vi "Load meas device config.vi"(7 "Equipo a Utilizar":enum16{"SR830 Lock In", "TDS 2012B Osciloscope"}(ring), 8 "error in (no error)":errorcluster, 10 "Datos Adquisición":T1={"Equipo a Utilizar"=enum."TDS 2012B Osciloscope", "Montura"=enum."Zaber T-LSR450B", "Datos Zaber"={"Sentido de Adquisición"=TRUE, "Comenzar Desde Home?"=TRUE, "Distancia a recorrer (um)"=10.0, "Pasos motor"=0, "Distancia entre Lecturas (um)"=0.1, "Puerto"="UNKNOWN"}, "Datos Bipolar/Unipolar"={"Puerto COM"="UNKNOWN", "Pasos entre Lecturas"=0, "Numero de lecturas"=0, "Sentido del motor"=TRUE}, "Datos Archivo"={"Ruta Archivo"=path "", "Nombre de Prueba"=""}, "Datos actuales"={"Montura"="", "Equipo"="", "Posición Actual"="", "Distancia Total a recorrer"="", "distancia Entre lecturas"="", "Pasos entre lecturas"=""}, "Datos a Guardar In"={"Datos Cursor Tektronix"="", "Datos Lokin"="", "Posición Cero"=0.0, "Posición Actual"=0.0}, "Datos Osciloscopio"={"Sesión Visa Osciloscopio"="UNKNOWN", "Tipo de Adquisición"=enum."Voltaje Pico Pico", "Canal a Utilizar"=enum."Canal 1", "Parametros de Adquisición"=enum."Una Muestra", "Número Promedio"=2}, "Datos Lock In"={"Visa Lock in"="Tektronix_TDS2012C"}} {"Datos Osciloscopio"."Número Promedio" min=2 max=20; "Datos a Guardar In"."Posición Actual" format="%#_10f"; "Datos a Guardar In"."Posición Cero" format="%#_10f"; "Datos Bipolar/Unipolar"."Numero de lecturas" max=910098 step=1}, 11 "Refnum in":T7) -> (0 "error out":errorcluster, 2 "Datos Adquisición out":T1={"Equipo a Utilizar"=enum."TDS 2012B Osciloscope", "Montura"=enum."Zaber T-LSR450B", "Datos Zaber"={"Sentido de Adquisición"=FALSE, "Comenzar Desde Home?"=FALSE, "Distancia a recorrer (um)"=0.0, "Pasos motor"=0, "Distancia entre Lecturas (um)"=0.0, "Puerto"=""}, "Datos Bipolar/Unipolar"={"Puerto COM"="", "Pasos entre Lecturas"=0, "Numero de lecturas"=0, "Sentido del motor"=TRUE}, "Datos Archivo"={"Ruta Archivo"=path "", "Nombre de Prueba"=""}, "Datos actuales"={"Montura"="", "Equipo"="", "Posición Actual"="", "Distancia Total a recorrer"="", "distancia Entre lecturas"="", "Pasos entre lecturas"=""}, "Datos a Guardar In"={"Datos Cursor Tektronix"="", "Datos Lokin"="", "Posición Cero"=0.0, "Posición Actual"=0.0}, "Datos Osciloscopio"={"Sesión Visa Osciloscopio"="Tektronix_TDS2012C", "Tipo de Adquisición"=enum."Voltaje Pico Pico", "Canal a Utilizar"=enum."Canal 1", "Parametros de Adquisición"=enum."Una Muestra", "Número Promedio"=2}, "Datos Lock In"={"Visa Lock in"="Tektronix_TDS2012C"}} {"Datos Osciloscopio"."Número Promedio" min=2 max=20; "Datos a Guardar In"."Posición Actual" format="%#_10f"; "Datos a Guardar In"."Posición Cero" format="%#_10f"; "Datos Bipolar/Unipolar"."Numero de lecturas" max=910098 step=1}, 3 "Refnum out":T7)   [LabVIEW 2020]
uses:
  Type Definitions/datos osciloscopio.ctl
  <vilib>/Utility/config.llb/NI_LVConfig.lvlib
  <vilib>/Utility/config.llb/Read Key (String).vi
  <vilib>/Utility/config.llb/Read Key (U32).vi
  <vilib>/Utility/config.llb/Read Key (I32).vi
  <vilib>/Utility/config.llb/Config Data RefNum.ctl
  Type Definitions/Datos Zaber.ctl
  Type Definitions/parametros motores.ctl
  Type Definitions/Datos a Guardar.ctl
  H:/Mi unidad/Departamento de Ingenieria/Investigadores/Gabriel Ramos/Proyecto Monturas v13/LV Source/Type Definitions/Tipos de montura.ctl
  Type Definitions/Asistente de adquisicion Cluster.ctl
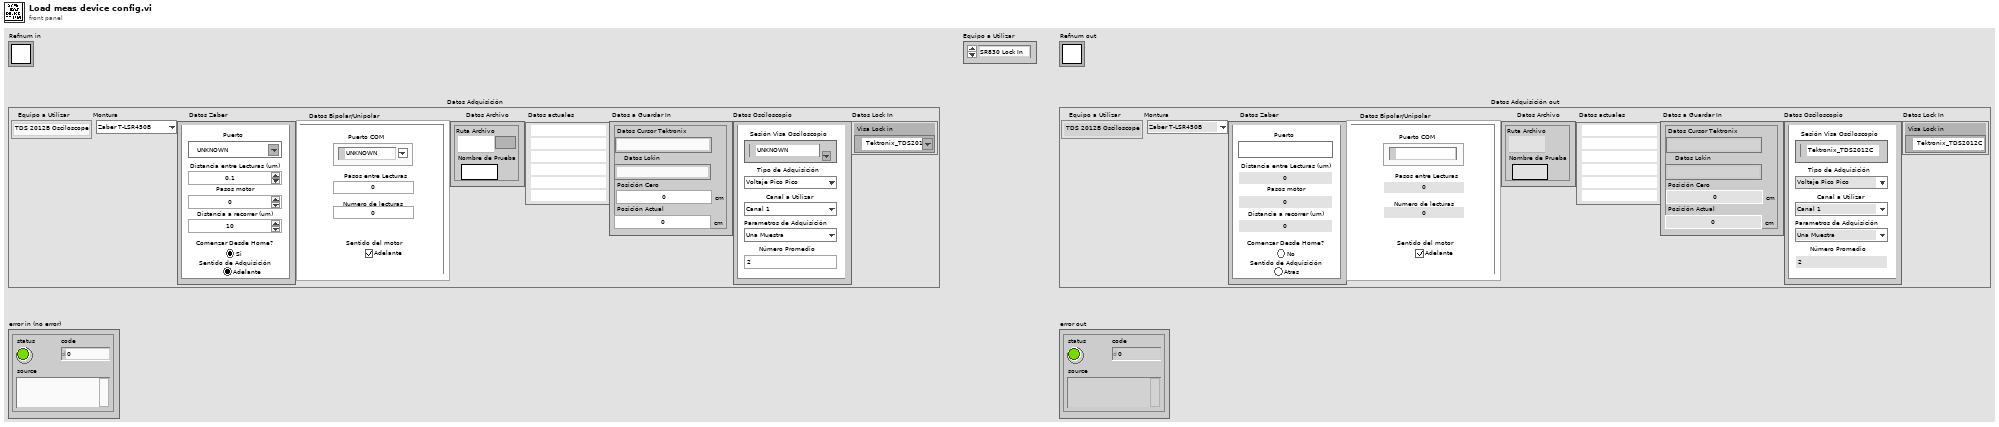
[diagram p1: front panel]
types:
  T1 = typedef "Asistente de adquisicion Cluster.ctl" = cluster{"Equipo a Utilizar":enum16{"SR830 Lock In", "TDS 2012B Osciloscope"}, "Montura":T2, "Datos Zaber":T3, "Datos Bipolar/Unipolar":T4, "Datos Archivo":cluster{"Ruta Archivo":path, "Nombre de Prueba":string}, "Datos actuales":cluster{"Montura":string, "Equipo":string, "Posición Actual":string, "Distancia Total a recorrer":string, "distancia Entre lecturas":string, "Pasos entre lecturas":string}, "Datos a Guardar In":T5, "Datos Osciloscopio":T6, "Datos Lock In":cluster{"Visa Lock in":refnum<visa-resource-name>}}
  T2 = typedef "Tipos de montura.ctl" = enum16{"Zaber T-LSR450B", "Zaber-T-LSR300B", "Zaber-T-LSRxxx", "Motor Bipolar", "Motor Unipolar"}
  T3 = typedef "Datos Zaber.ctl" = cluster{"Sentido de Adquisición":bool, "Comenzar Desde Home?":bool, "Distancia a recorrer (um)":dbl, "Pasos motor":i32, "Distancia entre Lecturas (um)":dbl, "Puerto":refnum<visa-resource-name>}
  T4 = typedef "parametros motores.ctl" = cluster{"Puerto COM":refnum<visa-resource-name>, "Pasos entre Lecturas":u16, "Numero de lecturas":u32, "Sentido del motor":bool}
  T5 = typedef "Datos a Guardar.ctl" = cluster{"Datos Cursor Tektronix":string, "Datos Lokin":string, "Posición Cero":dbl[unit], "Posición Actual":dbl[unit]}
  T6 = typedef "datos osciloscopio.ctl" = cluster{"Sesión Visa Osciloscopio":refnum<visa-resource-name>, "Tipo de Adquisición":enum16{"Voltaje Pico Pico", "Voltaje RMS", "Cursor Tiempo"}, "Canal a Utilizar":enum16{"Canal 1", "Canal 2", "Canal 1 y 2"}, "Parametros de Adquisición":enum16{"Una Muestra", "Promedio"}, "Número Promedio":i32}
  T7 = typedef "NI_LVConfig.lvlib/Config Data RefNum.ctl" = refnum<k1>
  T8 = cluster{"Visa Lock in":refnum<visa-resource-name>}
  T9 = enum16{"Voltaje Pico Pico", "Voltaje RMS", "Cursor Tiempo"}
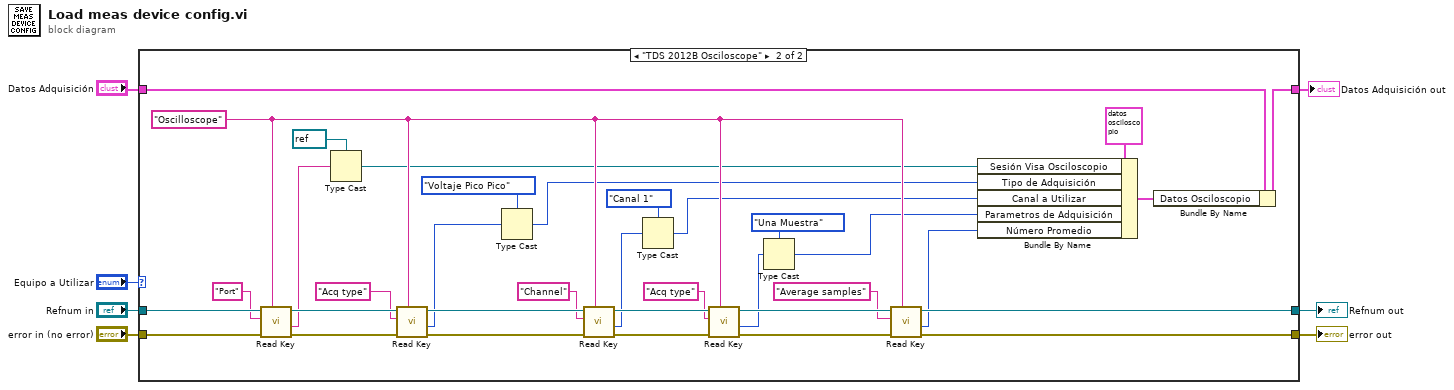
[diagram p0: block diagram]
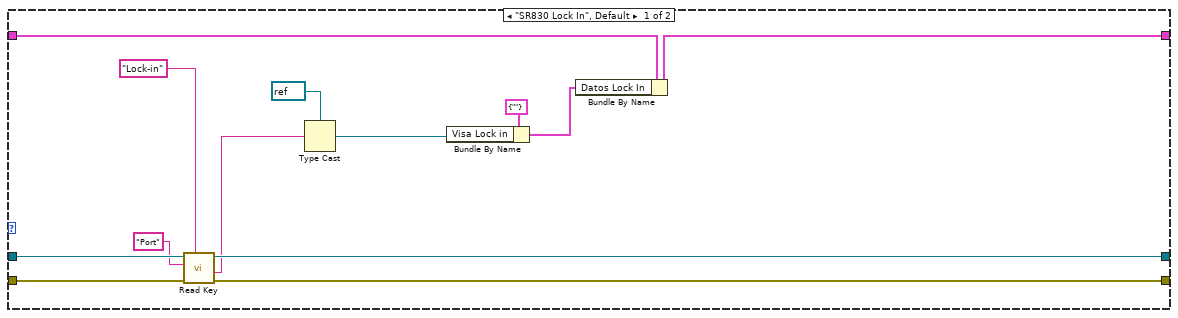
[diagram p2: hidden frame]
diagram:
  n1 = case shown="\"TDS 2012B Osciloscope\"" "Equipo a Utilizar" {
    tunnel: "error in (no error)" -> [w20 w55]
    tunnel: [w19 w42] -> w5
    tunnel: "Refnum in" -> [w18 w53]
    tunnel: [w17 w40] -> w7
    tunnel: "Datos Adquisición" -> [w10 w33]
    tunnel: [w8 w32] -> w1
    frame "SR830 Lock In", Default {
      n2 = call-poly <vilib>:"Read Key.vi"("section"="Lock-in", "error in (no error)"=w20, "key"="Port", "refnum"=w18) -> ("error out"=w19:errorcluster, "value"=w12:string, "refnum out"=w17:T7)  [unwired: 4 in, 1 out]
      n3 = Type Cast(type=refnum<visa-resource-name> refnum ("Visa Lock in"), x=w12) -> (*(type *) &x=w11:refnum<visa-resource-name>)
      n4 = Bundle By Name(cluster=T8 {"Visa Lock in"=""} ("Datos Lock In"), "Visa Lock in"=w11) -> (w9:T8)
      n5 = Bundle By Name(cluster=w10, "Datos Lock In"=w9) -> (w8:T1)
    }
    frame "TDS 2012B Osciloscope" {
      w39 = "Oscilloscope" ("section")
      n6 = call-poly <vilib>:"Read Key.vi"("section"=w39, "error in (no error)"=w55, "key"="Port", "refnum"=w53) -> ("error out"=w54:errorcluster, "value"=w36:string, "refnum out"=w50:T7)  [unwired: 4 in, 1 out]
      n7 = Type Cast(type=refnum<visa-resource-name> refnum ("Sesión Visa Osciloscopio"), x=w36) -> (*(type *) &x=w34:refnum<visa-resource-name>)
      n8 = call-poly <vilib>:"Read Key.vi"("section"=w39, "error in (no error)"=w54, "key"="Acq type", "refnum"=w50) -> ("error out"=w51:errorcluster, "value"=w29:u32, "refnum out"=w47:T7)  [unwired: 4 in, 1 out]
      n9 = Type Cast(type=T9."Voltaje Pico Pico" ("Tipo de Adquisición"), x=w29) -> (*(type *) &x=w28:T9)
      n10 = call-poly <vilib>:"Read Key.vi"("section"=w39, "error in (no error)"=w51, "key"="Channel", "refnum"=w47) -> ("error out"=w48:errorcluster, "value"=w26:u32, "refnum out"=w44:T7)  [unwired: 4 in, 1 out]
      n11 = Type Cast(type=enum16{"Canal 1", "Canal 2", "Canal 1 y 2"}."Canal 1" ("Canal a Utilizar"), x=w26) -> (*(type *) &x=w25:enum16{"Canal 1", "Canal 2", "Canal 1 y 2"})
      n12 = call-poly <vilib>:"Read Key.vi"("section"=w39, "error in (no error)"=w48, "key"="Acq type", "refnum"=w44) -> ("error out"=w45:errorcluster, "value"=w24:u32, "refnum out"=w41:T7)  [unwired: 4 in, 1 out]
      n13 = Type Cast(type=enum16{"Una Muestra", "Promedio"}."Una Muestra" ("Parametros de Adquisición"), x=w24) -> (*(type *) &x=w22:enum16{"Una Muestra", "Promedio"})
      n14 = call-poly <vilib>:"Read Key.vi"("section"=w39, "error in (no error)"=w45, "key"="Average samples", "refnum"=w41) -> ("error out"=w42:errorcluster, "value"=w21:i32, "refnum out"=w40:T7)  [unwired: 4 in, 1 out]
      n15 = Bundle By Name(cluster=T6 {"Sesión Visa Osciloscopio"="", "Tipo de Adquisición"=enum."Voltaje Pico Pico", "Canal a Utilizar"=enum."Canal 1", "Parametros de Adquisición"=enum."Una Muestra", "Número Promedio"=0} ("Datos Osciloscopio"), "Sesión Visa Osciloscopio"=w34, "Tipo de Adquisición"=w28, "Canal a Utilizar"=w25, "Parametros de Adquisición"=w22, "Número Promedio"=w21) -> (w31:T6)
      n16 = Bundle By Name(cluster=w33, "Datos Osciloscopio"=w31) -> (w32:T1)
    }
  }
  "Refnum out" <- w7
  "error out" <- w5
  "Datos Adquisición out" <- w1
